vi "xio.strip_lua.vi"(5 "LuaVIEW reference":T1) -> (15 "error out":errorcluster)   [LabVIEW 2012]
doc: "Returns the name of the last component of a path and the stripped path that leads up to that component.\nParameters:\nstr:path, path to strip\nResults:\nstr:stripped, path up to last component.\nstr:name, name of last component."
uses:
  typedefs/t_LuaVIEW Reference.ctl
  subvis/private/LuaVIEW Pull (path).vi
  subvis/private/LuaVIEW Push (path).vi
  subvis/private/LuaVIEW Push (string).vi
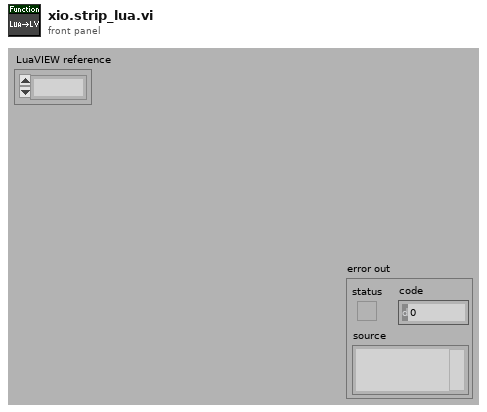
[diagram p1: front panel]
types:
  T1 = typedef "t_LuaVIEW Reference.ctl" = refnum<k1>
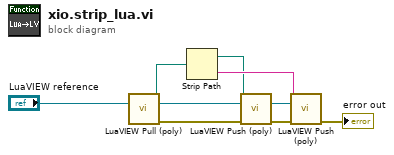
[diagram p0: block diagram]
diagram:
  n1 = call-poly "LuaVIEW Pull (poly).vi"("LuaVIEW reference in"="LuaVIEW reference") -> ("path"=w8:path, "LuaVIEW reference out"=w7:T1, "error out"=w5:errorcluster)  [unwired: 12 in]
  n2 = Strip Path(path=w8) -> (stripped path=w1:path, name=w2:string)
  n3 = call-poly "LuaVIEW Push (poly).vi"("path"=w1, "LuaVIEW reference in"=w7, "error in (no error)"=w5) -> ("LuaVIEW reference out"=w4:T1, "error out"=w6:errorcluster)  [unwired: 11 in]
  n4 = call-poly "LuaVIEW Push (poly).vi"("string"=w2, "LuaVIEW reference in"=w4, "error in (no error)"=w6) -> ("error out"=→"error out":errorcluster)  [unwired: 11 in, 1 out]
